vi "ConfigureTrigger.vi"(8 "error in (no error)":errorcluster, 9 "Simulation":T2, 10 "Trigger":T3={"Level"=0.04, "Source"=enum."Channel 2", "Slope"=enum."Rising", "mode"=enum."Single"} {"Level" format="%#_6p"}, 11 "picoscope in":refnum<class "picoscope.lvclass">) -> (0 "error out":errorcluster, 2 "Trigger":T3={"Level"=0.04, "Source"=enum."Channel 2", "Slope"=enum."Rising", "mode"=enum."Single"} {"Level" format="%#_6p"}, 3 "picoscope out":refnum<class "picoscope.lvclass">)   [LabVIEW 2020, in "picoscope.lvclass"]
uses:
  picoscope.lvclass
  trigger ctl.ctl
  OnOffTypeDef.ctl
  picoscope.lvclass/picoscope.ctl
panel:
  out "output cluster":T1
  in  "Trigger Settings":T1={"Trigger Enabled"=FALSE, "Trigger Source"=enum."Channel A", "Trigger Threshold (volts)"=0.0, "Trigger Direction"=2, "Trigger Delay (samples)"=0, "Auto Trigger Time (ms)"=1000} {"Trigger Direction" items=["Rising"=2, "Falling"=3]}
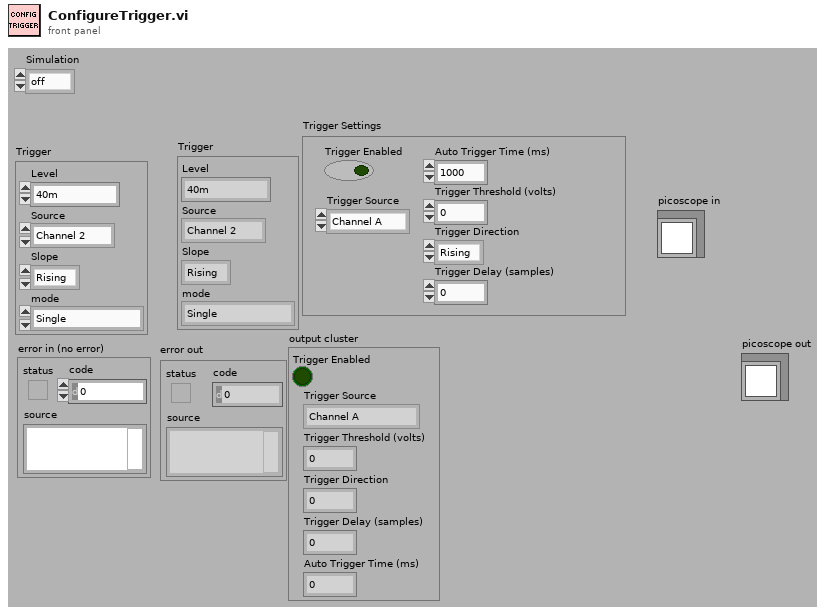
[diagram p1: front panel]
types:
  T1 = cluster{"Trigger Enabled":bool, "Trigger Source":enum16{"Channel A", "Channel B", "Channel C", "Channel D", "Ext."}, "Trigger Threshold (volts)":dbl, "Trigger Direction":u16, "Trigger Delay (samples)":u32, "Auto Trigger Time (ms)":i16}
  T2 = typedef "OnOffTypeDef.ctl" = enum16{"off", "on"}
  T3 = typedef "trigger ctl.ctl" = cluster{"Level":dbl, "Source":enum16{"Channel 1", "Channel 2", "Channel 3", "Channel 4", "External", "Power Line"}, "Slope":enum16{"Rising", "Falling"}, "mode":enum16{"Auto", "Normal", "Single", "Single auto trigger"}}
  T4 = enum16{"Channel 1", "Channel 2", "Channel 3", "Channel 4", "External", "Power Line"}
  T5 = enum16{"Auto", "Normal", "Single", "Single auto trigger"}
  T6 = cluster{"Enabled":bool, "Coupling":i16, "Range":u16, "Analogue Offset":sgl}
  T7 = cluster{"Driver Version":string, "USB Version":string, "Hardware":string, "Variant":string, "Batch and Serial":string, "Cal Date":string, "Kernel Version":string, "Digital HW Version":string, "Analogue HW Version":string, "MSO":bool, "Number of channels":i16}
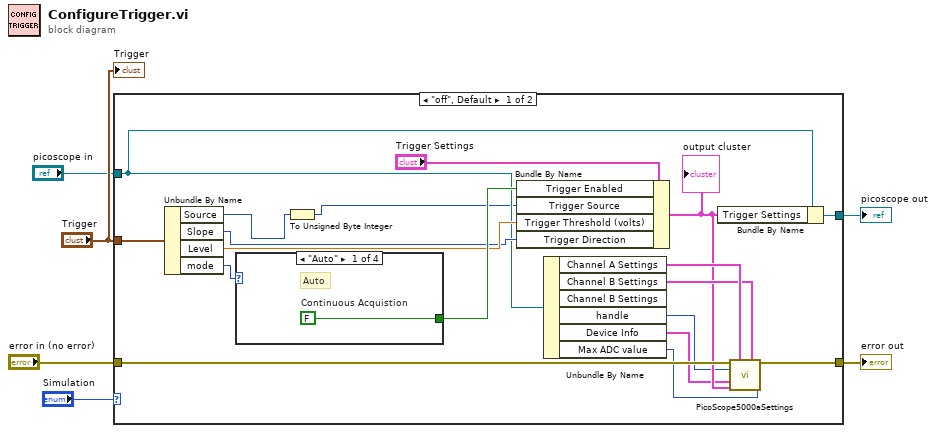
[diagram p0: block diagram]
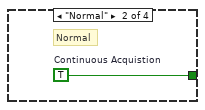
[diagram p2: hidden frame]
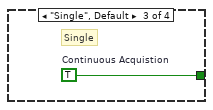
[diagram p3: hidden frame]
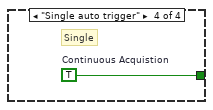
[diagram p4: hidden frame]
diagram:
  n1 = case shown="\"off\", Default" "Simulation" {
    tunnel: [w14 w30] -> w6
    tunnel: "Trigger" -> [w23 _]
    tunnel: "error in (no error)" -> [w13 w30]
    tunnel: "picoscope in" -> [w16 w29]
    tunnel: [w15 w29] -> w1
    frame "off", Default {
      n2 = Unbundle By Name(w23) -> ("Source"=w8:T4, "Slope"=w17:enum16{"Rising", "Falling"}, "Level"=w18:dbl, "mode"=w24:T5)
      n3 = case shown="\"Auto\"" w24 {
        tunnel: [w25 w26 w27 w28] -> w19
        frame "Auto" {
          w25 = FALSE  # Continuous Acquistion
          # "Auto"
        }
        frame "Normal" {
          w26 = TRUE  # Continuous Acquistion
          # "Normal"
        }
        frame "Single", Default {
          w27 = TRUE  # Continuous Acquistion
          # "Single"
        }
        frame "Single auto trigger" {
          w28 = TRUE  # Continuous Acquistion
          # "Single"
        }
      }
      n4 = To Unsigned Byte Integer(number=w8) -> (unsigned 8bit integer=w7:u8)
      n5 = Bundle By Name(cluster="Trigger Settings", "Trigger Enabled"=w19, "Trigger Source"=w7, "Trigger Threshold (volts)"=w18, "Trigger Direction"=w17) -> (w12:T1)
      "output cluster" <- w12
      n6 = Unbundle By Name(w16) -> ("Channel A Settings"=w22:T6, "Channel B Settings"=w21:T6, "handle"=w11:i16, "Device Info"=w10:T7, "Max ADC value"=w9:i16)  [unwired: 1 out]
      n7 = Bundle By Name(cluster=w16, "Trigger Settings"=w12) -> (w15:refnum<class "picoscope.lvclass">)
      n8 = call "PicoScope5000aSettings.vi"("error in"=w13, "Channel A Settings"=w22, "Channel B Settings"=w21, "handle in"=w11, "Device Info"=w10, "Trigger Settings"=w12, "Max ADC value"=w9) -> ("error out"=w14:errorcluster)  [unwired: 6 in, 2 out]
    }
    frame "on" {
      # "Simulation Mode ON"
    }
  }
  "error out" <- w6
  "picoscope out" <- w1
  "Trigger" <- "Trigger"
